vi "ReadTemps.vi"(8 "error in (no error)":errorcluster, 11 "reference in":refnum<class "Flux_Capacitor.lvclass">) -> (0 "error out":errorcluster, 1 "Real":dbl[](array[numeric]), 2 "Raw":i32[](array[numeric]), 3 "reference in":refnum<class "Flux_Capacitor.lvclass">)   [LabVIEW 2022 SP3, in "Flux_Capacitor.lvlib" / "Flux_Capacitor.lvclass"]
uses:
  Flux_Capacitor.lvclass
  <vilib>/numeric/Random Number (Range) U64.vi
  <vilib>/numeric/sub_Random U32.vi
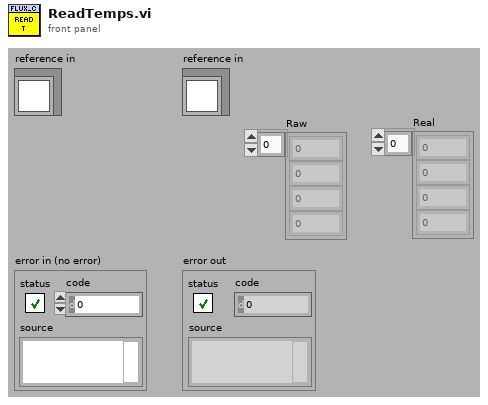
[diagram p1: front panel]
types:
  T1 = typedef "Flux_Capacitor.lvlib/Flux_Capacitor.lvclass/ObjectAttributes.ctl" = cluster{"Config":T2, "T Sensors":T3[], "Temp_DegC":dbl[], "Temp_Raw":u64[], "RTC":timestamp, "Flux":bool, "Time":timestamp, "RTC_Live":timestamp}
  T2 = typedef "Flux_Capacitor.lvlib/Flux_Capacitor.lvclass/Config.ctl" = cluster{"default":string}
  T3 = typedef "Flux_Capacitor.lvlib/Flux_Capacitor.lvclass/TempSensor.ctl" = enum16{"1", "2", "3"}
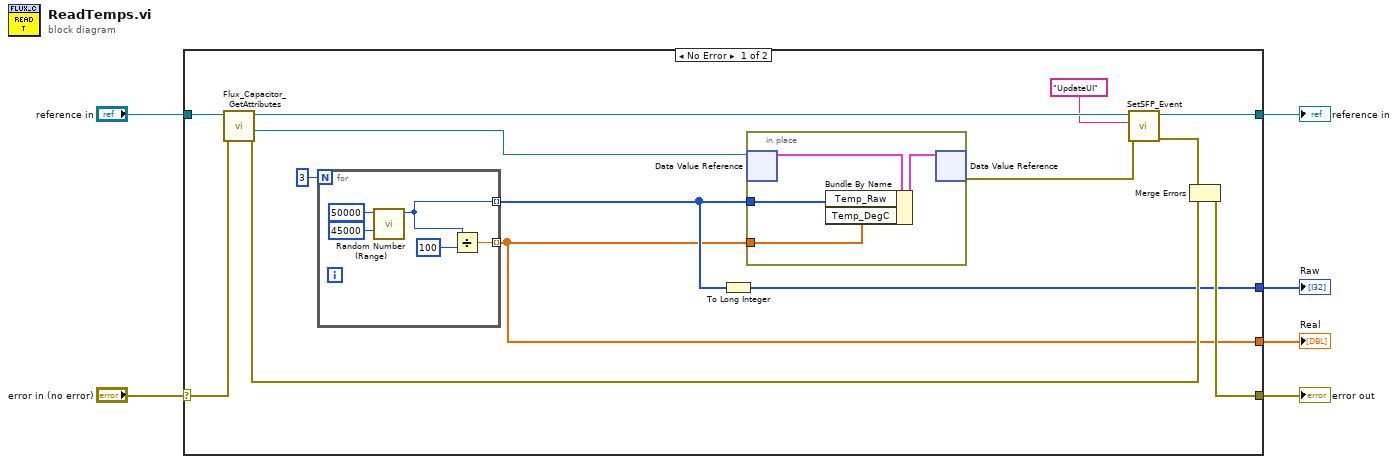
[diagram p0: block diagram]
diagram:
  n1 = case shown="No Error" "error in (no error)" {
    selector: "error in (no error)" -> [w20 w31]
    tunnel: [w10 w31] -> w4
    tunnel: [w14 w30] -> w3
    tunnel: "reference in" -> [w19 w30]
    tunnel: [w8 _] -> w2
    tunnel: [w7 _] -> w1
    frame No Error {
      n2 = call "Flux_Capacitor_GetAttributes.vi"("error in (no error)"=w20, "reference in"=w19) -> ("error out"=w12:errorcluster, "DataRef"=w18:refnum<data-value>, "reference out"=w16:refnum<class "Flux_Capacitor.lvclass">)  [unwired: 6 in, 1 out]
      n3 = for {
        N: 3 -> [_]
        tunnel: [w21] -> w7 mode=indexing
        tunnel: [w23] -> w9 mode=indexing
        n4 = call-poly <vilib>:"Random Number (Range).vi"("lower bound (0)"=u64 45000, "upper bound (100)"=u64 50000) -> ("number"=w23:u64)  [unwired: 9 in]
        n5 = Divide(x=w23, y=u64 100) -> (x/y=w21:dbl)
      }
      n6 = To Long Integer(number=w9) -> (32bit integer=w8:i32[])
      n7 = in-place {
        in-place-border: w9 -> [w28]
        in-place-border: w7 -> [w27]
        n8 = in-place-dvr #1(w18) -> (w29:T1)  [unwired: 1 out]
        n9 = Bundle By Name(cluster=w29, "Temp_Raw"=w28, "Temp_DegC"=w27) -> (w26:T1)
        n10 = in-place-dvr #1(w26) -> (w13:errorcluster)  [unwired: 1 out]
      }
      n11 = call-dynamic "SetSFP_Event.vi"("error in (no error)"=w13, "msg"="UpdateUI", "reference in"=w16) -> ("error out"=w11:errorcluster, "reference out"=w14:refnum<class "Flux_Capacitor.lvclass">)  [unwired: 7 in]
      n12 = Merge Errors(w11, w12) -> (w10:errorcluster)
    }
    frame Error {
    }
  }
  "error out" <- w4
  "reference in" <- w3
  "Raw" <- w2
  "Real" <- w1
